vi "国弘滤波次数设置.vi"(7 "探头":u16(ring)=5 items=["NULL", "pH", "Cond", "DO", "Turb", "ORP", "6", "7", "8", "9", "氯化物"], 8 "error in (no error)":errorcluster caption="错误输入（无错误）", 11 "滤波次数":u16) -> (0 "error out":errorcluster caption="错误输出", 3 "MB session out":refnum<class "MB_Master.lvclass">)   [LabVIEW 2016, in "斯坦道多参数.lvlib"]
uses:
  <vilib>/Plasmionique/MB Master/MB_Master/MB_Master.lvclass
  <vilib>/Plasmionique/MB Master/MB Master.lvlib
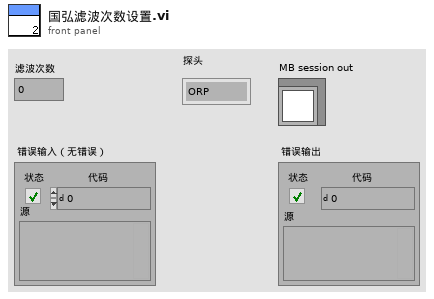
[diagram p1: front panel]
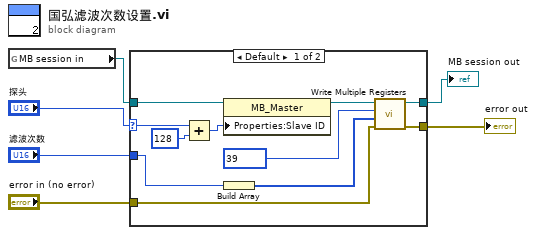
[diagram p0: block diagram]
diagram:
  n1 = global read "多参数全局变量.vi" "MB session in"() -> (w1:refnum<class "MB_Master.lvclass">)
  n2 = case shown="Default" "探头" {
    selector: "探头" -> [w9 _]
    tunnel: "error in (no error)" -> [w16 w18]
    tunnel: "滤波次数" -> [w8 _]
    tunnel: w1 -> [w12 w19]
    tunnel: [w11 w18] -> w4
    tunnel: [w10 w19] -> w3
    frame Default {
      n3 = Add(x=w9, y=u16 128) -> (x+y=w15:u16)
      n4 = property class="MB_Master"(reference=w12, "Properties:Slave ID"=w15) -> (reference out=w13:refnum<class "MB_Master.lvclass">)  [unwired: 1 in, 1 out]
      n5 = Build Array(w8) -> (w7:u16[])
      n6 = call <vilib>:"Write Multiple Registers.vi"("error in (no error)"=w16, "values"=w7, "starting address"=u16 39, "MB session in"=w13) -> ("error out"=w11:errorcluster, "MB session out"=w10:refnum<class "MB_Master.lvclass">)  [unwired: 6 in]
    }
    frame 0 {
    }
  }
  "error out" <- w4
  "MB session out" <- w3
